vi "DevelopTest.vi"() -> ()   [LabVIEW 2020]
panel:
  out "Boolean 2":bool
  out "Boolean":bool
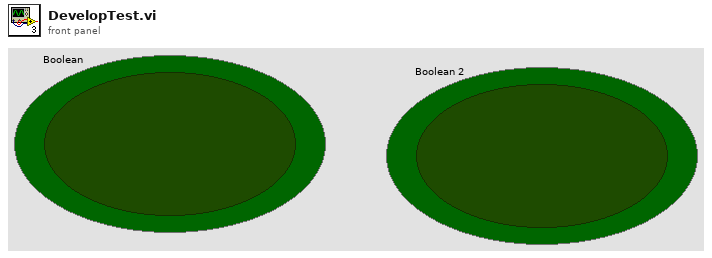
[diagram p1: front panel]
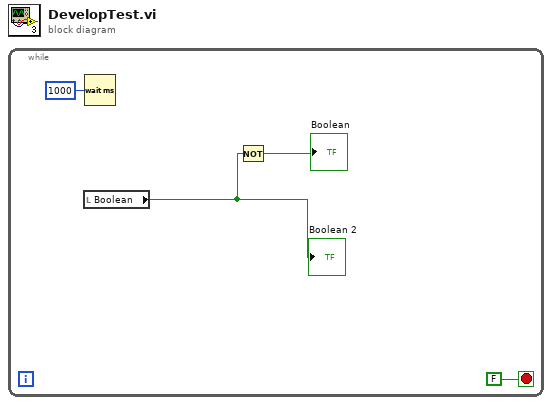
[diagram p0: block diagram]
diagram:
  n1 = while {
    stop <- FALSE stop-if-true
    n2 = local read "Boolean"() -> (w2:bool)
    "Boolean 2" <- w2
    n3 = Wait (ms)(milliseconds to wait=u32 1000) -> ()  [unwired: 1 out]
    n4 = Not(x=w2) -> (.not. x?=→"Boolean":bool)
  }
